vi "prompt_with_timeout_v1.0.vi"(9 "timer(sec)":i32=-1, 10 "message in":string="Current setup condition(s):\n\n1. Oven temperature: 45 Deg C\n2. Relative Humidity: 67%", 11 "title in":string="Confirm/Acknowldege Start of Test") -> ()   [LabVIEW 2025]
doc: "Use this template to build a producer/consumer design pattern with events to produce queue items. Use this design pattern instead of the User Interface Event Handler pattern for user interfaces when you want to execute code asynchronously in response to an event without slowing the user interface responsiveness."
panel:
  out "consumer_exit":bool
  out "message":string
  out "title":string
  out "timeout_msg":string
  in  "cancel":bool
  in  "confirm":bool
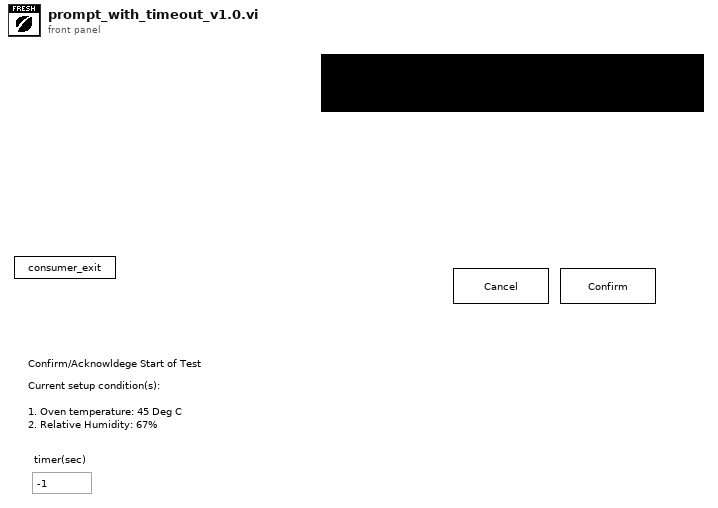
[diagram p1: front panel]
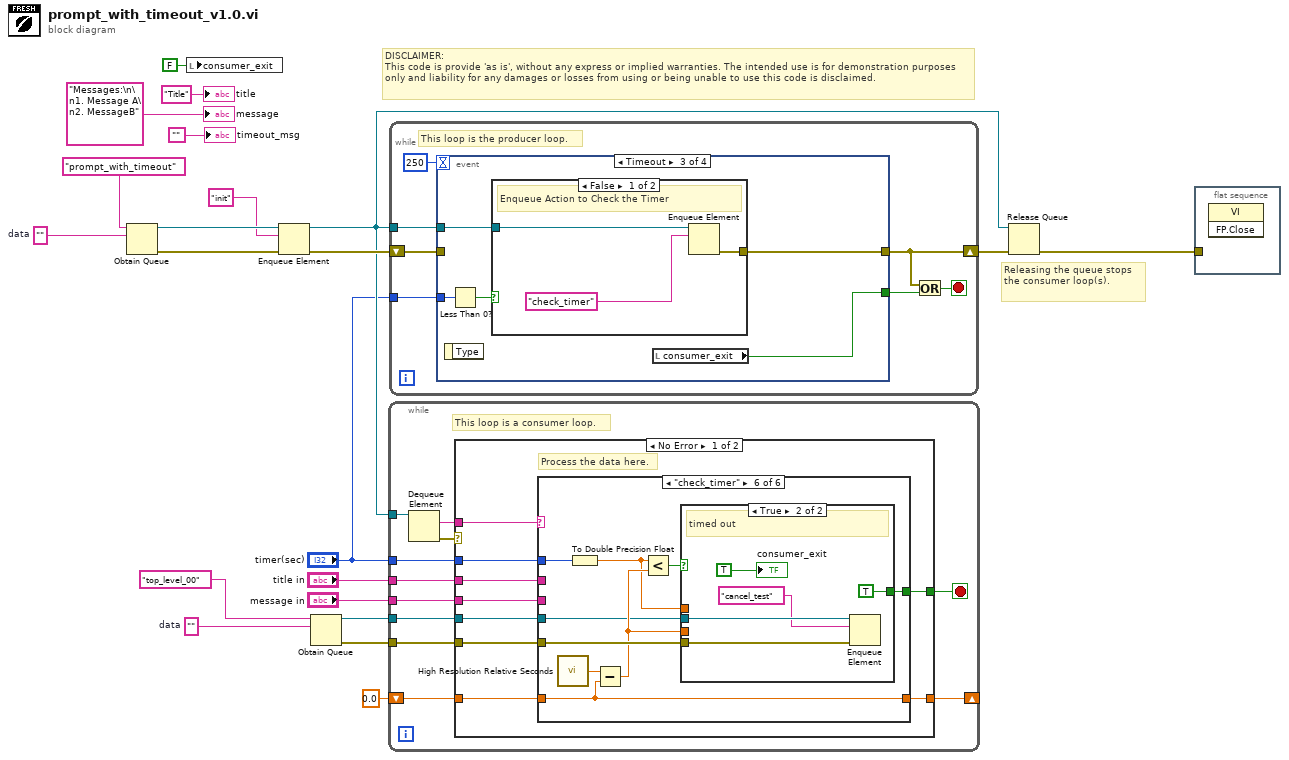
[diagram p0: block diagram]
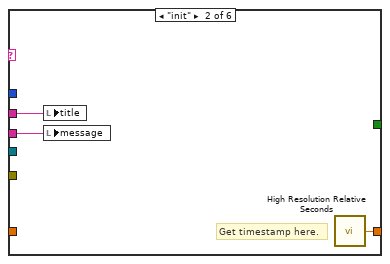
[diagram p3: hidden frame]
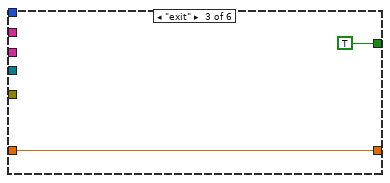
[diagram p4: hidden frame]
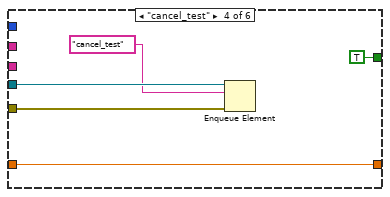
[diagram p5: hidden frame]
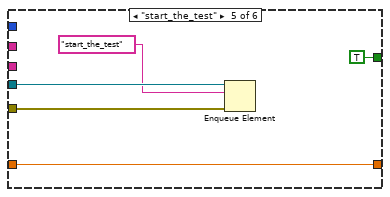
[diagram p6: hidden frame]
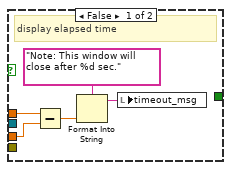
[diagram p7: hidden frame]
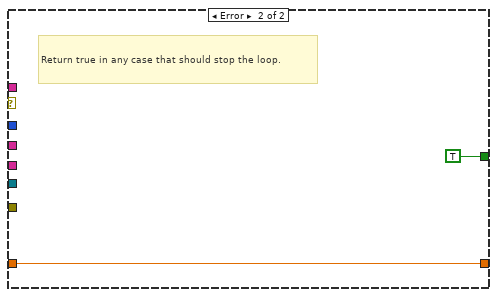
[diagram p8: hidden frame]
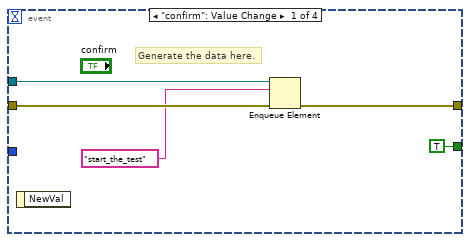
[diagram p9: hidden frame]
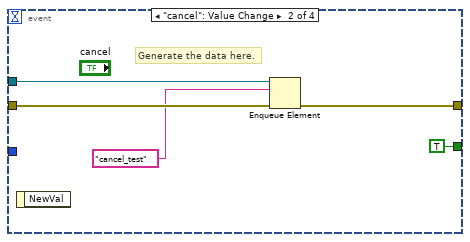
[diagram p10: hidden frame]
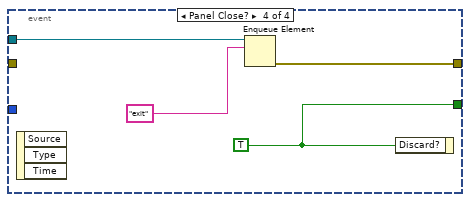
[diagram p12: hidden frame]
diagram:
  w2 = ""  # data
  w4 = ""  # data
  # "DISCLAIMER:\nThis code is provide 'as is', without any express or implied warranties. The intended use is for demonstration purposes only and liability for any damages or losses from using or being unable to use this code is disclaimed."
  # "Releasing the queue stops the consumer loop(s)."
  n1 = Obtain Queue(name (unnamed)="prompt_with_timeout", element data type=w4) -> (queue out=w11:refnum<queue>, error out=w14:errorcluster)  [unwired: 3 in, 1 out]
  n2 = local write "consumer_exit"(FALSE ("consumer_exit")) -> ()
  n3 = Enqueue Element(queue=w11, element="init" ("action"), error in (no error)=w14) -> (queue out=w12:refnum<queue>, error out=w13:errorcluster)  [unwired: 1 in, 1 out]
  n4 = Obtain Queue(name (unnamed)="top_level_00", element data type=w2) -> (queue out=w6:refnum<queue>, error out=w15:errorcluster)  [unwired: 3 in, 1 out]
  n5 = while {
    tunnel: w12 -> [w32]
    tunnel: w15 -> [w28]
    shift-right: [w27] -> _
    shift-left: 0.0 ("relative seconds") -> [w26]
    tunnel: "title in" -> [w25]
    tunnel: "message in" -> [w24]
    tunnel: "timer(sec)" -> [w23]
    tunnel: w6 -> [w22]
    stop <- w29 stop-if-true
    # "This loop is a consumer loop."
    n6 = Dequeue Element(queue=w32) -> (element=w30:string, error out=w31:errorcluster)  [unwired: 2 in, 2 out]
    n7 = case shown="No Error" w31 {
      tunnel: w30 -> [w33 _]
      tunnel: [w41 TRUE] -> w29
      tunnel: w28 -> [w40 _]
      tunnel: [w39 w77] -> w27
      tunnel: w26 -> [w38 w77]
      tunnel: w25 -> [w37 _]
      tunnel: w24 -> [w36 _]
      tunnel: w23 -> [w35 _]
      tunnel: w22 -> [w34 _]
      frame No Error {
        # "Process the data here."
        n8 = case shown="\"check_timer\"" w33 {
          tunnel: [_ _ TRUE TRUE TRUE w59] -> w41
          tunnel: w40 -> [_ _ _ w52 w57 w66]
          tunnel: [w42 w45 w46 w51 w56 w64] -> w39
          tunnel: w38 -> [w42 _ w46 w51 w56 w64]
          tunnel: w37 -> [_ w44 _ _ _ _]
          tunnel: w36 -> [_ w43 _ _ _ _]
          tunnel: w35 -> [_ _ _ _ _ w62]
          tunnel: w34 -> [_ _ _ w50 w55 w60]
          frame Default {
          }
          frame "init" {
            # "Get timestamp here."
            n9 = local write "title"(w44) -> ()
            n10 = local write "message"(w43) -> ()
            n11 = call <vilib>:"High Resolution Relative Seconds.vi"() -> ("relative seconds"=w45:dbl)
          }
          frame "exit" {
          }
          frame "cancel_test" {
            n12 = Enqueue Element(queue=w50, element="cancel_test", error in (no error)=w52) -> ()  [unwired: 1 in, 3 out]
          }
          frame "start_the_test" {
            n13 = Enqueue Element(queue=w55, element="start_the_test", error in (no error)=w57) -> ()  [unwired: 1 in, 3 out]
          }
          frame "check_timer" {
            n14 = call <vilib>:"High Resolution Relative Seconds.vi"() -> ("relative seconds"=w65:dbl)
            n15 = To Double Precision Float(number=w62) -> (double precision float=w58:dbl)
            n16 = Subtract(x=w65, y=w64) -> (x-y=w61:dbl)
            n17 = Less?(x=w58, y=w61) -> (x < y?=w63:bool)
            n18 = case shown="True" w63 {
              tunnel: w66 -> [_ w76]
              tunnel: w61 -> [w68 _]
              tunnel: w60 -> [_ w75]
              tunnel: [_ TRUE] -> w59
              tunnel: w58 -> [w69 _]
              frame False {
                # "display elapsed time"
                n19 = Subtract(x=w69, y=w68) -> (x-y=w67:dbl)
                n20 = Format Into String(format string="Note: This window will close after %d sec.", w67) -> (resulting string=w71:string)  [unwired: 2 in, 1 out]
                n21 = local write "timeout_msg"(w71) -> ()
              }
              frame True {
                # "timed out"
                n22 = Enqueue Element(queue=w75, element="cancel_test", error in (no error)=w76) -> ()  [unwired: 1 in, 3 out]
                "consumer_exit" <- TRUE ("consumer_exit")
              }
            }
          }
        }
      }
      frame Error {
        # "Return true in any case that should stop the loop."
      }
    }
  }
  n23 = while {
    shift-right: [w81] -> w21
    shift-left: w13 -> [w84]
    tunnel: w12 -> [w85]
    tunnel: "timer(sec)" -> [w79]
    stop <- w82 stop-if-true
    # "This loop is the producer loop."
    n24 = event shown="[2] Timeout" {
      selector: _ -> [_ _ _ _]
      dyn-events: _ -> [_ _ _ _]
      timeout: 250 -> [_ _ _ _]
      tunnel: w85 -> [w90 w95 w99 w106]
      tunnel: w84 -> [w89 w94 _ _]
      tunnel: [w88 w93 w100 w107] -> w81
      tunnel: [TRUE ("Discard?") TRUE ("Discard?") w96 w105] -> w83
      tunnel: w79 -> [_ _ w98 _]
      event "confirm": Value Change {
        # "Generate the data here."
        n25 = event-data() -> ()  [unwired: 1 in, 1 out]
        n26 = Enqueue Element(queue=w90, element="start_the_test", error in (no error)=w89) -> (error out=w88:errorcluster)  [unwired: 1 in, 2 out]
      }
      event "cancel": Value Change {
        # "Generate the data here."
        n27 = event-data() -> ()  [unwired: 1 in, 1 out]
        n28 = Enqueue Element(queue=w95, element="cancel_test", error in (no error)=w94) -> (error out=w93:errorcluster)  [unwired: 1 in, 2 out]
      }
      event Timeout {
        n29 = event-data() -> ()  [unwired: 1 in, 1 out]
        n30 = Less Than 0?(x=w98) -> (x < 0?=w97:bool)
        n31 = case shown="False" w97 {
          tunnel: [w103 _] -> w100
          tunnel: w99 -> [w102 _]
          frame False {
            # "Enqueue Action to Check the Timer"
            n32 = Enqueue Element(queue=w102, element="check_timer") -> (error out=w103:errorcluster)  [unwired: 2 in, 2 out]
          }
          frame True {
          }
        }
        n33 = local read "consumer_exit"() -> (w96:bool)
      }
      event Panel Close? {
        w105 = TRUE ("Discard?")
        n34 = event-data() -> ()  [unwired: 1 in, 3 out]
        n35 = Enqueue Element(queue=w106, element="exit") -> (error out=w107:errorcluster)  [unwired: 2 in, 2 out]
        n36 = event-data("Discard?"=w105) -> ()  [unwired: 1 in, 1 out]
      }
    }
    n37 = Or(x=w81, y=w83) -> (x .or. y?=w82:bool)
  }
  n38 = Release Queue(queue=w12, error in (no error)=w21) -> (error out=w5:errorcluster)  [unwired: 1 in, 2 out]
  n39 = flat-sequence {
    tunnel: w5 -> [_]
    frame #0 {
      n40 = invoke class="VI" method="FP.Close"() -> ()  [unwired: 3 in, 3 out]
    }
  }
  "timeout_msg" <- ""
  "title" <- "Title" ("title")
  "message" <- "Messages:\n\n1. Message A\n2. MessageB" ("message")
